vi "Trial.vi"(2 "error in (no error)":errorcluster, 3 "queue in":refnum<queue>, 4 "DDA":bool=TRUE) -> (0 "error out":errorcluster, 1 "queue out":refnum<queue>)   [LabVIEW 2017]
uses:
  Control/RPY.ctl
  <vilib>/Analysis/baseanly.llb/Real Dot Product.vi
  <vilib>/Analysis/_algsub.llb/Real Vector Norm.vi
  <vilib>/Analysis/baseanly.llb/Outer Product.vi
  <vilib>/Analysis/baseanly.llb/Real Outer Product.vi
  <vilib>/robotics/Kinematics/Create Lie Group Matrix.vi
  Global.vi
  <vilib>/Analysis/7linalg.llb/Create Special Matrix.vi
  <vilib>/Analysis/7linalg.llb/Create Special Real Matrix.vi
  <vilib>/Analysis/Matrix/Numeric/Multiply/Multiply.vi
  <vilib>/Analysis/Matrix/Numeric/Multiply/Multiply - RM,R.vi
  <vilib>/Analysis/Matrix/Numeric/Multiply/Multiply - R,RM.vi
  <vilib>/Analysis/Matrix/Numeric/Add/Add.vi
  <vilib>/Analysis/Matrix/Numeric/Add/Add - RM,RM.vi
  <vilib>/Analysis/NI_AALPro.lvlib
  <vilib>/robotics/Kinematics/NI_Kinematics.lvlib
  Control/Damping.ctl
  <vilib>/Analysis/NI_AALBase.lvlib
panel:
  in  "alpha theta":dbl=0.1
  in  "alpha w":dbl=0.1
  in  "lambda theta":dbl=0.9
  in  "lambda w":dbl=0.9
  in  "alpha Rbar":dbl=0.1
  in  "RoM (deg)":dbl=75.0 format="%#_13g"
  in  "Weber's Rule":dbl[](array[numeric])=[1.2, 1.0, 0.8]
  in  "n x(s, a)":i32=3
  in  "n x(s)":i32=3
  in  "Variable":T1
  in  "Time Target (s)":dbl=5.0
  in  "epsilon":dbl=0.1
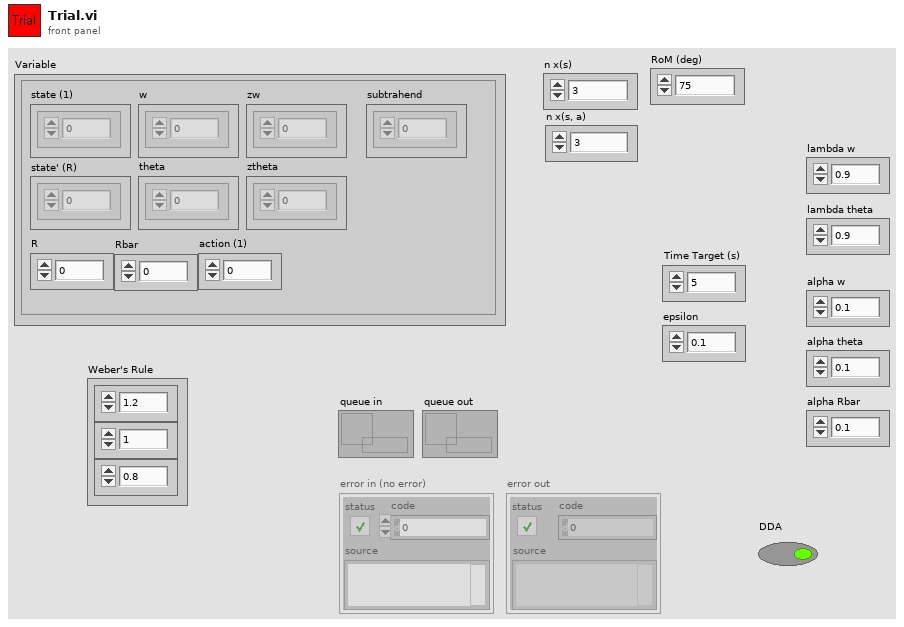
[diagram p1: front panel]
types:
  T1 = cluster{"w":dbl[], "theta":dbl[], "state (1)":dbl[], "state' (R)":dbl[], "R":dbl, "Rbar":dbl, "zw":dbl[], "ztheta":dbl[], "action (1)":dbl, "subtrahend":dbl[]}
  T2 = typedef "RPY.ctl" = cluster{"roll":dbl, "pitch":dbl, "yaw":dbl}
  T3 = typedef "Damping.ctl" = cluster{"Cx":dbl, "Cy":dbl, "Cz":dbl}
  T4 = typedef "NI_Matrix.lvlib/RealMatrix.ctl" = dbl[][]
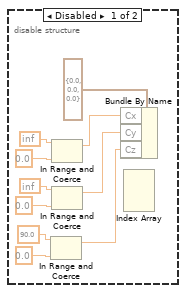
[diagram p2: hidden frame]
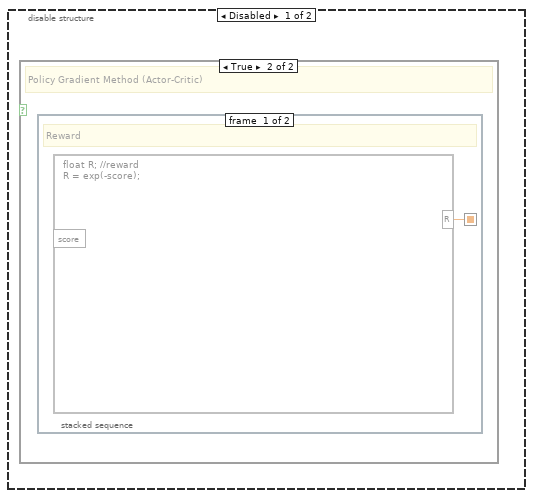
[diagram p3: hidden frame]
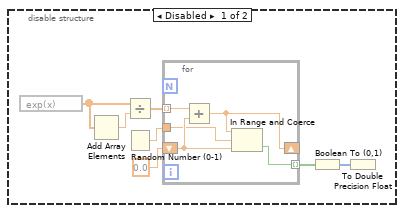
[diagram p6: hidden frame]
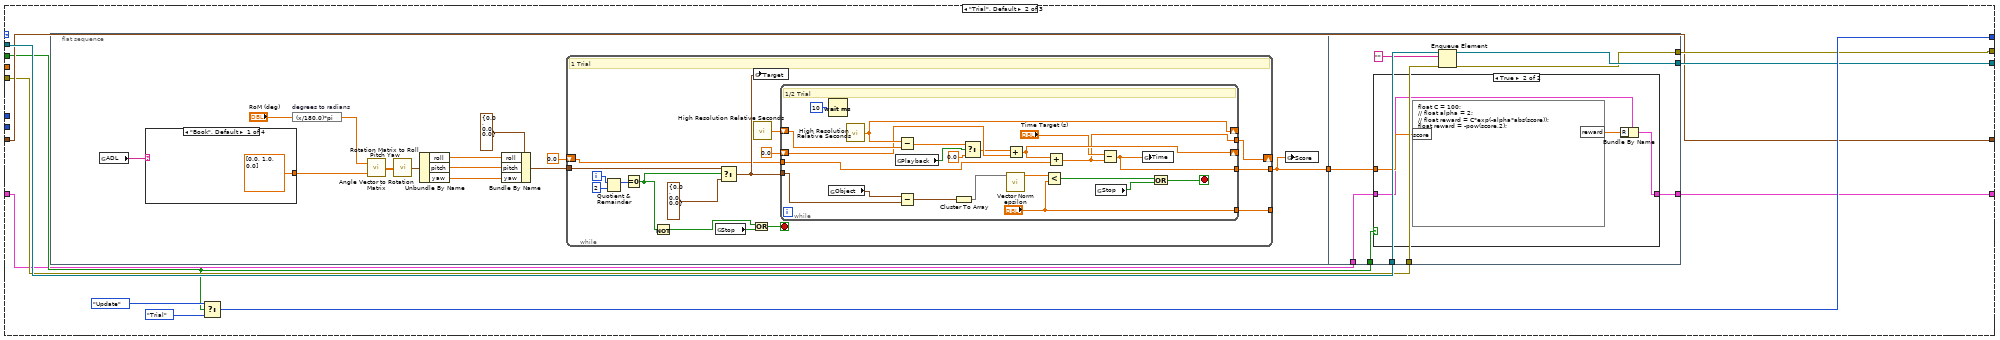
[diagram p7: hidden frame]
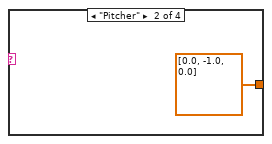
[diagram p8: hidden frame]
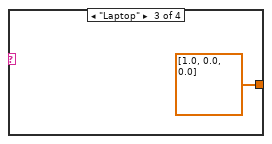
[diagram p9: hidden frame]
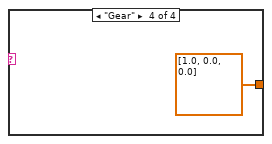
[diagram p10: hidden frame]
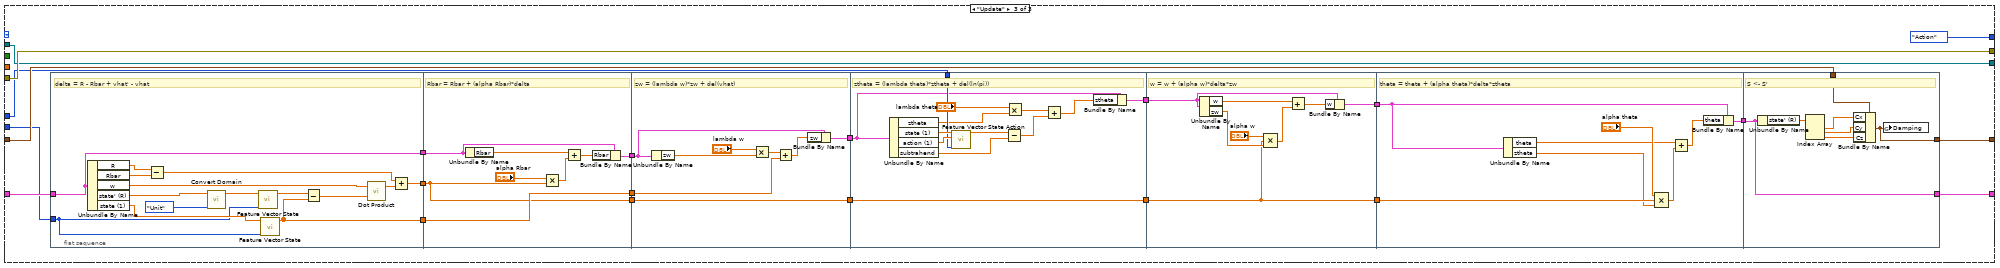
[diagram p12: hidden frame]
diagram:
  n1 = flat-sequence {
    tunnel: "error in (no error)" -> [w16]
    tunnel: "queue in" -> [w18]
    tunnel: "DDA" -> [w11]
    tunnel: [w17] -> w2
    tunnel: [w15] -> w1
    frame #0 {
      n2 = flat-sequence {
        tunnel: [w35] -> w9
        tunnel: ["n x(s, a)"] -> w8
        tunnel: [w32] -> w7
        tunnel: ["n x(s)"] -> w6
        frame #0 {
          w33 = 3
          n3 = for {
            N: w33 -> [_]
            tunnel: [w38] -> w32 mode=concatenating
            tunnel: w33 -> [w37]
            tunnel: w33 -> [w36]
            i -> [w39]
            n4 = for {
              N: w37 -> [_]
              tunnel: w39 -> [w43]
              tunnel: [w41] -> w38 mode=concatenating
              tunnel: w36 -> [w40]
              i -> [w42]
              n5 = for {
                N: w40 -> [_]
                tunnel: w43 -> [w50]
                tunnel: w42 -> [w49]
                tunnel: [w44] -> w41 mode=indexing
                i -> [w48]
                n6 = Index Array(array="Weber's Rule", index #1=w50, index #2=w49, index #3=w48) -> (element #1=w47:dbl, element #2=w46:dbl, element #3=w45:dbl)
                n7 = Build Array(w47, w46, w45) -> (w44:dbl[])
              }
            }
          }
          n8 = call "Feature Vector State Action.vi"("n x(s, a)"="n x(s, a)", "action"=0.0, "state"=dbl[] [0.0, 0.0, 0.0]) -> ("x(s, a)"=w30:dbl[])  [unwired: 8 in]
          n9 = call "Feature Vector State.vi"("n x(s)"="n x(s)", "state"=dbl[] [0.0, 0.0, 0.0]) -> ("x(s)"=w23:dbl[])  [unwired: 9 in]
          n10 = Array Size(array=w23) -> (size(s)=w24:i32)
          n11 = Array Size(array=w30) -> (size(s)=w29:i32)
          n12 = Initialize Array(0.0 ("element"), w24) -> (w20:dbl[])
          n13 = Initialize Array(0.0 ("element"), w29) -> (w19:dbl[])
          n14 = Bundle By Name(cluster="Variable", "w"=w20, "zw"=w20, "theta"=w19, "ztheta"=w19) -> (w35:T1)
        }
      }
      n15 = Select(t=enum16{"Action", "Trial", "Update"}."Action", s=w11, f=enum16{"Action", "Trial", "Update"}."Trial") -> (s? t:f=w12:enum16{"Action", "Trial", "Update"})
      n16 = global read "Global.vi" "Damping"() -> (w10:T3)
      n17 = while {
        shift-right: [w60] -> w17
        shift-left: w18 -> [w62]
        shift-right: [w59] -> w15
        shift-left: w16 -> [w61]
        shift-right: [w64] -> _
        shift-left: w12 -> [w65]
        tunnel: w11 -> [w63]
        shift-right: [w57] -> _
        shift-left: w10 -> [w58]
        shift-right: [w53] -> _
        shift-left: w9 -> [w56]
        tunnel: w8 -> [w55]
        tunnel: w7 -> [w54]
        tunnel: w6 -> [w52]
        stop <- w66 stop-if-true
        # "State Machine"
        n18 = case shown="\"Action\"" w65 {
          tunnel: [enum16{"Action", "Trial", "Update"}."Trial" w131 enum16{"Action", "Trial", "Update"}."Action"] -> w64
          tunnel: w63 -> [_ w124 _]
          tunnel: w62 -> [w94 w130 w221]
          tunnel: w61 -> [w95 w125 w222]
          tunnel: [w94 w129 w221] -> w60
          tunnel: [w95 w128 w222] -> w59
          tunnel: w58 -> [w93 w126 w212]
          tunnel: [w93 w126 w211] -> w57
          tunnel: w56 -> [w81 w123 w218]
          tunnel: w55 -> [w86 _ w206]
          tunnel: w54 -> [w85 _ _]
          tunnel: [w79 w122 w213] -> w53
          tunnel: w52 -> [_ _ w210]
          frame "Action" {
            w91 = 27
            n19 = Unbundle By Name(w81) -> ("theta"=w90:dbl[])
            n20 = Cluster To Array(cluster=w93) -> (array=w83:dbl[])
            n21 = call "Convert Domain.vi"("Direction"=enum16{"Unit", "Real"}."Unit", "Real"=w83) -> ("Unit"=w82:dbl[])  [unwired: 9 in]
            n22 = To Double Precision Float(number=w91) -> (double precision float=w75:dbl)
            n23 = Bundle By Name(cluster=w81, "state (1)"=w82) -> (w80:T1)
            n24 = for {
              N: w91 -> [_]
              tunnel: w75 -> [w120]
              tunnel: w82 -> [w116]
              tunnel: w90 -> [w115]
              tunnel: [w114] -> w89 mode=indexing
              tunnel: w86 -> [w113]
              tunnel: [w112] -> w71 mode=indexing
              i -> [w119]
              n25 = To Double Precision Float(number=w119) -> (double precision float=w118:dbl)
              n26 = Divide(x=w118, y=w120) -> (x/y=w117:dbl)
              n27 = call "Feature Vector State Action.vi"("n x(s, a)"=w113, "action"=w117, "state"=w116) -> ("x(s, a)"=w112:dbl[])  [unwired: 8 in]
              n28 = call-poly <vilib>:"Dot Product.vi"("Y Vector"=w112, "X Vector"=w115) -> ("X * Y"=w114:dbl)  [unwired: 1 out]
            }
            n29 = Index Array(array=w71) -> (element=w70:dbl[])  [unwired: 2 in]
            n30 = Array Size(array=w70) -> (size(s)=w69:i32)
            n31 = flat-sequence {
              tunnel: w89 -> [w111]
              tunnel: [w110] -> w73
              frame #0 {
                # "Softmax"
                n32 = Exponential(1:w111) -> (0:w109:dbl[])
                n33 = Add Array Elements(numeric array=w109) -> (sum=w108:dbl)
                n34 = Divide(x=w109, y=w108) -> (x/y=w110:dbl[])
              }
            }
            n35 = Initialize Array(0.0 ("element"), w69) -> (w67:dbl[])
            n36 = for {
              tunnel: w73 -> [w101] mode=indexing
              tunnel: w71 -> [w100] mode=indexing
              shift-right: [w97] -> w72
              shift-left: w67 -> [w99]
              # "sigma(pi(a|s, theta)*x(s, a))"
              n37 = Multiply(x=w101, y=w100) -> (x*y=w98:dbl[])
              n38 = Add(x=w98, y=w99) -> (x+y=w97:dbl[])
            }
            n39 = Random Number (0-1)() -> (number: 0 to 1=w87:dbl)
            n40 = for {
              tunnel: w73 -> [w106] mode=indexing
              shift-right: [w104] -> _
              shift-left: 0.0 -> [w105]
              tunnel: w87 -> [w107]
              tunnel: [w102] -> w77
              i -> [w102]
              stop <- w103 stop-if-true
              n41 = Add(x=w106, y=w105) -> (x+y=w104:dbl)
              n42 = In Range and Coerce(upper limit=w104, x=w107, lower limit=w105) -> (In Range?=w103:bool)  [unwired: 1 out]
            }
            n43 = Index Array(array=w85, index (row)=w77) -> (element=w84:dbl[])  [unwired: 1 in]
            n44 = To Double Precision Float(number=w77) -> (double precision float=w76:dbl)
            n45 = Multiply(x=w83, y=w84) -> (x*y=w78:dbl[])
            n46 = Divide(x=w76, y=w75) -> (x/y=w74:dbl)
            n47 = Bundle By Name(cluster=w80, "state' (R)"=w78, "action (1)"=w74, "subtrahend"=w72) -> (w79:T1)
          }
          frame "Trial", Default {
            n48 = flat-sequence {
              tunnel: [w133] -> w121
              tunnel: w130 -> [w196]
              tunnel: [w195] -> w129
              tunnel: [w194] -> w128
              tunnel: w125 -> [w192]
              tunnel: w124 -> [w191]
              tunnel: [w189] -> w122
              tunnel: w123 -> [w190]
              tunnel: w121 -> [w188]
              frame #0 {
                n49 = global read "Global.vi" "ADL"() -> (w137:string)
                n50 = case shown="\"Book\", Default" w137 {
                  tunnel: [dbl[] [0.0, 1.0, 0.0] dbl[] [0.0, -1.0, 0.0] dbl[] [1.0, 0.0, 0.0] dbl[] [1.0, 0.0, 0.0]] -> w136
                  frame "Book", Default {
                  }
                  frame "Pitcher" {
                  }
                  frame "Laptop" {
                  }
                  frame "Gear" {
                  }
                }
                n51 = expression code="(x/180.0)*pi" "degrees to radians"("RoM (deg)") -> (w134:dbl)
                n52 = call <vilib>:"Angle Vector to Rotation Matrix.vi"("vector"=w136, "angle"=w134) -> ("rotation matrix"=w140:T4)
                n53 = call <vilib>:"Rotation Matrix to Roll Pitch Yaw.vi"("rotation matrix"=w140) -> ("angles"=w141:cluster{"roll":dbl, "pitch":dbl, "yaw":dbl})
                n54 = Unbundle By Name(w141) -> ("roll"=w142:dbl, "pitch"=w143:dbl, "yaw"=w144:dbl)
                n55 = Bundle By Name(cluster=T2 {"roll"=0.0, "pitch"=0.0, "yaw"=0.0} ("Target"), "roll"=w142, "pitch"=w143, "yaw"=w144) -> (w138:T2)
                n56 = while {
                  tunnel: w138 -> [w160]
                  shift-right: [w152] -> _
                  shift-left: 0.0 -> [w153]
                  tunnel: [w151] -> _
                  tunnel: [w150] -> w133
                  i -> [w163]
                  stop <- w156 stop-if-true
                  # "1 Trial"
                  n57 = Quotient & Remainder(x=w163, y=2) -> (x-y*floor(x/y)=w161:i32)  [unwired: 1 out]
                  n58 = Equal To 0?(x=w161) -> (x = 0?=w155:bool)
                  n59 = Not(x=w155) -> (.not. x?=w154:bool)
                  n60 = global read "Global.vi" "Stop"() -> (w157:bool)
                  n61 = Select(t=w160, s=w155, f=T2 {"roll"=0.0, "pitch"=0.0, "yaw"=0.0} ("Target")) -> (s? t:f=w158:T2)
                  n62 = Or(x=w154, y=w157) -> (x .or. y?=w156:bool)
                  n63 = global write "Global.vi" "Target"(w158) -> ()
                  n64 = call <vilib>:"High Resolution Relative Seconds.vi"() -> ("relative seconds"=w165:dbl)
                  n65 = while {
                    tunnel: w158 -> [w172]
                    shift-right: [w178] -> _
                    shift-left: w165 -> [w179]
                    shift-right: [w170] -> _
                    shift-left: 0.0 -> [w177]
                    tunnel: w153 -> [w171]
                    tunnel: [w168] -> w152
                    tunnel: ["epsilon"] -> w151
                    tunnel: [w166] -> w150
                    stop <- w180 stop-if-true
                    # "1/2 Trial"
                    n66 = Wait (ms)(milliseconds to wait=u32 10) -> ()  [unwired: 1 out]
                    n67 = global read "Global.vi" "Object"() -> (w185:T2)
                    n68 = call <vilib>:"High Resolution Relative Seconds.vi"() -> ("relative seconds"=w178:dbl)
                    n69 = global read "Global.vi" "Playback"() -> (w176:bool)
                    n70 = Subtract(x=w178, y=w179) -> (x-y=w175:dbl)
                    n71 = Subtract(x=w185, y=w172) -> (x-y=w186:T2)
                    n72 = Cluster To Array(cluster=w186) -> (array=w187:dbl[])
                    n73 = Select(t=w175, s=w176, f=0.0) -> (s? t:f=w174:dbl)
                    n74 = call-poly <vilib>:"Vector Norm.vi"("Input Vector"=w187) -> ("norm"=w184:dbl)  [unwired: 9 in, 1 out]
                    n75 = Add(x=w174, y=w177) -> (x+y=w170:dbl)
                    n76 = Less?(x=w184, y="epsilon") -> (x < y?=w183:bool)
                    n77 = Add(x=w170, y=w171) -> (x+y=w168:dbl)
                    n78 = global read "Global.vi" "Stop"() -> (w182:bool)
                    n79 = Subtract(x="Time Target (s)", y=w168) -> (x-y=w166:dbl)
                    n80 = global write "Global.vi" "Time"(w166) -> ()
                    n81 = Or(x=w183, y=w182) -> (x .or. y?=w180:bool)
                  }
                }
                n82 = global write "Global.vi" "Score"(w133) -> ()
              }
              frame #1 {
                n83 = case shown="True" w191 {
                  tunnel: w190 -> [w197 w200]
                  tunnel: [w197 w198] -> w189
                  tunnel: w188 -> [_ w201]
                  frame False {
                  }
                  frame True {
                    n84 = formula code="float C = 100;\n// float alpha = 2;\n// float reward = C*exp(-alpha*abs(score));\nfloat reward = -pow(score,2);"("score"=w201) -> ("reward"=w199:dbl)
                    n85 = Bundle By Name(cluster=w200, "R"=w199) -> (w198:T1)
                  }
                }
                n86 = Enqueue Element(queue=w196, element="", error in (no error)=w192) -> (queue out=w195:refnum<queue>, error out=w194:errorcluster)  [unwired: 1 in, 1 out]
              }
            }
            n87 = Select(t=enum16{"Action", "Trial", "Update"}."Update", s=w124, f=enum16{"Action", "Trial", "Update"}."Trial") -> (s? t:f=w131:enum16{"Action", "Trial", "Update"})
          }
          frame "Update" {
            n88 = flat-sequence {
              tunnel: [w238] -> w219
              tunnel: w218 -> [w238]
              tunnel: w210 -> [w231]
              tunnel: [w225] -> w209
              tunnel: [w224] -> w207
              tunnel: [w241] -> w220
              tunnel: w219 -> [w243]
              tunnel: w209 -> [w239]
              tunnel: [w240] -> w208
              tunnel: w207 -> [w240]
              tunnel: [w239] -> w203
              tunnel: w220 -> [w251]
              tunnel: [w249] -> w216
              tunnel: w208 -> [w248]
              tunnel: [w247] -> w204
              tunnel: w203 -> [w247]
              tunnel: [w256] -> w217
              tunnel: w216 -> [w258]
              tunnel: w206 -> [w265]
              tunnel: [w255] -> w205
              tunnel: w204 -> [w255]
              tunnel: w217 -> [w271]
              tunnel: [w269] -> w214
              tunnel: w205 -> [w268]
              tunnel: [w268] -> w202
              tunnel: [w276] -> w215
              tunnel: w214 -> [w277]
              tunnel: w202 -> [w282]
              tunnel: [w290] -> w213
              tunnel: w215 -> [w290]
              tunnel: w212 -> [w288]
              tunnel: [w284] -> w211
              frame #0 {
                # "delta = R - Rbar + vhat' - vhat"
                n89 = Unbundle By Name(w238) -> ("R"=w237:dbl, "Rbar"=w236:dbl, "w"=w228:dbl[], "state' (R)"=w234:dbl[], "state (1)"=w235:dbl[])
                n90 = Subtract(x=w237, y=w236) -> (x-y=w227:dbl)
                n91 = call "Convert Domain.vi"("Direction"=enum16{"Unit", "Real"}."Unit", "Real"=w234) -> ("Unit"=w232:dbl[])  [unwired: 9 in]
                n92 = call "Feature Vector State.vi"("n x(s)"=w231, "state"=w232) -> ("x(s)"=w230:dbl[])  [unwired: 9 in]
                n93 = call "Feature Vector State.vi"("n x(s)"=w231, "state"=w235) -> ("x(s)"=w224:dbl[])  [unwired: 9 in]
                n94 = Subtract(x=w230, y=w224) -> (x-y=w229:dbl[])
                n95 = call-poly <vilib>:"Dot Product.vi"("Y Vector"=w229, "X Vector"=w228) -> ("X * Y"=w226:dbl)  [unwired: 1 out]
                n96 = Add(x=w227, y=w226) -> (x+y=w225:dbl)
              }
              frame #1 {
                # "Rbar = Rbar + (alpha Rbar)*delta"
                n97 = Unbundle By Name(w243) -> ("Rbar"=w246:dbl)
                n98 = Multiply(x="alpha Rbar", y=w239) -> (x*y=w245:dbl)
                n99 = Add(x=w246, y=w245) -> (x+y=w242:dbl)
                n100 = Bundle By Name(cluster=w243, "Rbar"=w242) -> (w241:T1)
              }
              frame #2 {
                # "zw = (lambda w)*zw + del(vhat)"
                n101 = Unbundle By Name(w251) -> ("zw"=w254:dbl[])
                n102 = Multiply(x="lambda w", y=w254) -> (x*y=w252:dbl[])
                n103 = Add(x=w252, y=w248) -> (x+y=w250:dbl[])
                n104 = Bundle By Name(cluster=w251, "zw"=w250) -> (w249:T1)
              }
              frame #3 {
                # "ztheta = (lambda theta)*ztheta + del(ln(pi))"
                n105 = Unbundle By Name(w258) -> ("ztheta"=w262:dbl[], "state (1)"=w267:dbl[], "action (1)"=w266:dbl, "subtrahend"=w263:dbl[])
                n106 = call "Feature Vector State Action.vi"("n x(s, a)"=w265, "action"=w266, "state"=w267) -> ("x(s, a)"=w264:dbl[])  [unwired: 8 in]
                n107 = Subtract(x=w264, y=w263) -> (x-y=w259:dbl[])
                n108 = Multiply(x="lambda theta", y=w262) -> (x*y=w260:dbl[])
                n109 = Add(x=w260, y=w259) -> (x+y=w257:dbl[])
                n110 = Bundle By Name(cluster=w258, "ztheta"=w257) -> (w256:T1)
              }
              frame #4 {
                # "w = w + (alpha w)*delta*zw"
                n111 = Unbundle By Name(w271) -> ("w"=w275:dbl[], "zw"=w273:dbl[])
                n112 = Compound Arithmetic op=MULTIPLY("alpha w", w268, w273) -> (w272:dbl[])
                n113 = Add(x=w275, y=w272) -> (x+y=w270:dbl[])
                n114 = Bundle By Name(cluster=w271, "w"=w270) -> (w269:T1)
              }
              frame #5 {
                # "theta = theta + (alpha theta)*delta*ztheta"
                n115 = Unbundle By Name(w277) -> ("theta"=w279:dbl[], "ztheta"=w281:dbl[])
                n116 = Compound Arithmetic op=MULTIPLY("alpha theta", w282, w281) -> (w280:dbl[])
                n117 = Add(x=w279, y=w280) -> (x+y=w278:dbl[])
                n118 = Bundle By Name(cluster=w277, "theta"=w278) -> (w276:T1)
              }
              frame #6 {
                # "S <- S'"
                n119 = Unbundle By Name(w290) -> ("state' (R)"=w289:dbl[])
                n120 = Index Array(array=w289) -> (element #1=w287:dbl, element #2=w286:dbl, element #3=w285:dbl)  [unwired: 3 in]
                n121 = Bundle By Name(cluster=w288, "Cx"=w287, "Cy"=w286, "Cz"=w285) -> (w284:T3)
                n122 = global write "Global.vi" "Damping"(w284) -> ()
              }
            }
          }
        }
        n123 = global read "Global.vi" "Stop"() -> (w66:bool)
      }
    }
  }
  n124 = disable-structure shown="Enabled" {
    frame Disabled {
      n125 = In Range and Coerce(upper limit=90.0, lower limit=0.0) -> (coerced(x)=w300:dbl)  [unwired: 1 in, 1 out]
      n126 = In Range and Coerce(upper limit=inf, lower limit=0.0) -> (coerced(x)=w298:dbl)  [unwired: 1 in, 1 out]
      n127 = In Range and Coerce(upper limit=inf, lower limit=0.0) -> (coerced(x)=w299:dbl)  [unwired: 1 in, 1 out]
      n128 = Bundle By Name(cluster=T3 {"Cx"=0.0, "Cy"=0.0, "Cz"=0.0} ("State"), "Cx"=w298, "Cy"=w299, "Cz"=w300) -> ()  [unwired: 1 out]
      n129 = Index Array() -> ()  [unwired: 4 in, 3 out]
    }
    frame Enabled {
    }
  }
  n130 = disable-structure shown="Enabled" {
    frame Disabled {
      n131 = expression code="exp(x)"() -> (w303:dbl[])  [unwired: 1 in]
      n132 = Add Array Elements(numeric array=w303) -> (sum=w304:dbl)
      n133 = Divide(x=w303, y=w304) -> (x/y=w301:dbl[])
      n134 = Random Number (0-1)() -> (number: 0 to 1=w305:dbl)
      n135 = for {
        shift-right: [w311] -> _
        shift-left: 0.0 -> [w312]
        tunnel: w305 -> [w310]
        tunnel: [w309] -> w306 mode=indexing
        tunnel: w301 -> [w308] mode=indexing
        n136 = Add(x=w308, y=w312) -> (x+y=w311:dbl)
        n137 = In Range and Coerce(upper limit=w311, x=w310, lower limit=w312) -> (In Range?=w309:bool)  [unwired: 1 out]
      }
      n138 = Boolean To (0,1)(Boolean=w306) -> (0, 1=w307:i16[])
      n139 = To Double Precision Float(number=w307) -> ()  [unwired: 1 out]
    }
    frame Enabled {
    }
  }
  n140 = disable-structure shown="Enabled" {
    frame Disabled {
      n141 = case shown="True" {
        selector: _ -> [_ _]
        frame False {
        }
        frame True {
          # "Policy Gradient Method (Actor-Critic)"
          n142 = stacked-sequence {
            seq-local: [w313 _] -> [_ _]
            frame #0 {
              # "Reward"
              n143 = formula code="float R; //reward\nR = exp(-score);"() -> ("R"=w313:dbl)  [unwired: 1 in]
            }
            frame #1 {
            }
          }
        }
      }
    }
    frame Enabled {
    }
  }
  "error out" <- w1
  "queue out" <- w2
